vi "PieSesToAusPh.vi"(3 "error out":errorcluster, 4 "sinc":waveform(i16), 5 "Array":waveform(i16)[][](array[waveform])) -> ()   [LabVIEW 2010]
uses:
  <vilib>/Waveform/WDTOps.llb/WDT Append Waveforms DBL.vi
panel:
  out "A":i16[](array[numeric])
  out "us":sgl[](array[numeric]) format="%#.1f"
  out "size(s)":i32
  in  "index":i32
  out "Channel":string
  out "Waveform Graph":waveform(dbl)[](graph)
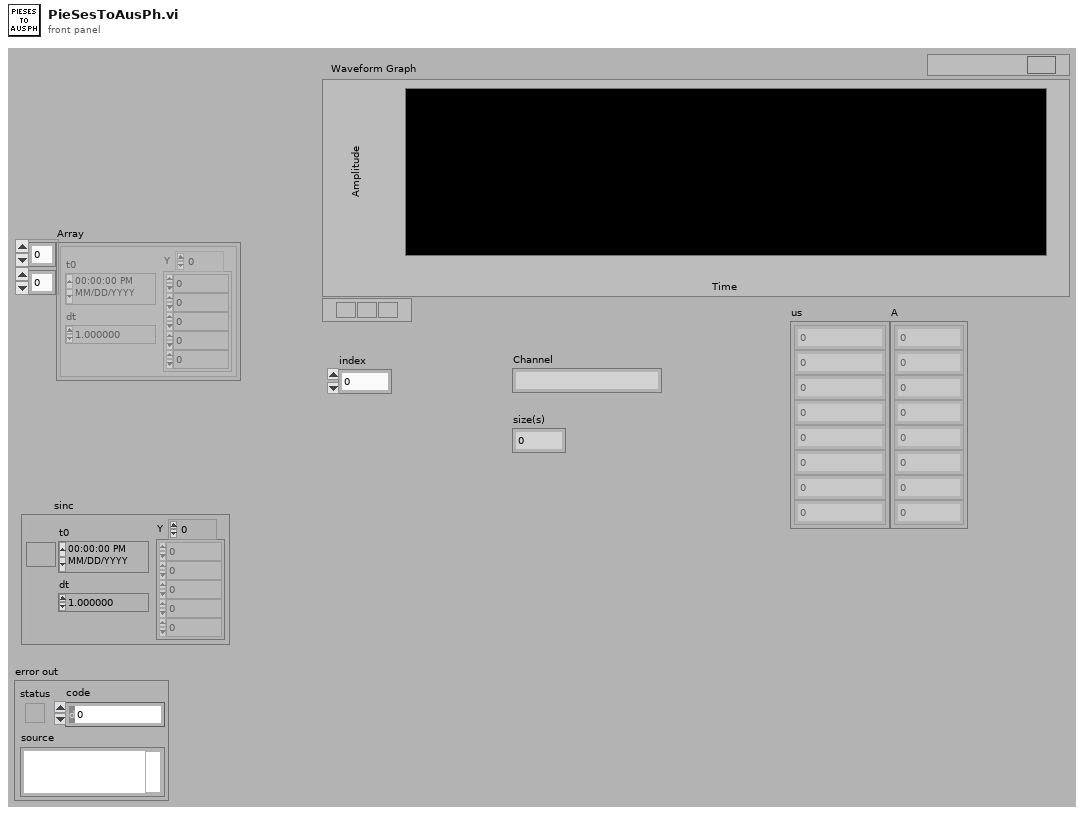
[diagram p1: front panel]
types:
  T1 = typedef "LVDateTimeRec.ctl" = cluster{"fractional second":dbl, "second":i32, "minute":i32, "hour":i32, "day of month":i32, "month":i32, "year":i32, "day of week":i32, "day of year":i32, "DST":i32}
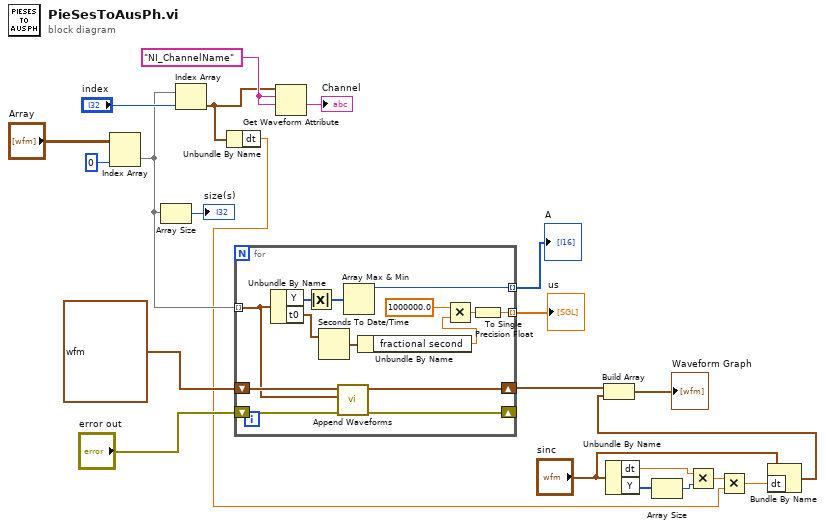
[diagram p0: block diagram]
diagram:
  w21 = "NI_ChannelName" ("name")
  n1 = Index Array(array="Array", index (col)=0 ("index (row)")) -> (element=w16:waveform(i16)[])  [unwired: 1 in]
  n2 = Array Size(array=w16) -> (size(s)=→"size(s)":i32)
  n3 = Index Array(array=w16, index="index") -> (element=w9:waveform(i16))
  n4 = Unbundle By Name(w9) -> ("dt"=w4:dbl)
  n5 = for {
    tunnel: w16 -> [w32] mode=indexing
    shift-right: [w36] -> _
    shift-left: "error out" -> [w35]
    shift-right: [w34] -> w11
    shift-left: waveform(dbl) {"t0"=timestamp(0 s since 1904-01-01), "dt"=1.0, "Y"=[]} ("waveform out") -> [w33]
    tunnel: [w29] -> w12 mode=indexing
    tunnel: [w26] -> w13 mode=indexing
    n6 = Unbundle By Name(w32) -> ("Y"=w31:i16[], "t0"=w28:timestamp)
    n7 = Absolute Value(x=w31) -> (abs(x)=w30:i16[])
    n8 = Seconds To Date/Time(time stamp (now)=w28) -> (date time rec=w27:T1)  [unwired: 1 in]
    n9 = call-poly <vilib>:"Append Waveforms.vi"("error in (no error)"=w35, "waveform B"=w32, "waveform A"=w33) -> ("error out"=w36:errorcluster, "waveform out"=w34:waveform(dbl))  [unwired: 7 in]
    n10 = Array Max & Min(array=w30) -> (max value=w29:i16)  [unwired: 3 out]
    n11 = Unbundle By Name(w27) -> ("fractional second"=w24:dbl)
    n12 = Multiply(x=1000000.0, y=w24) -> (x*y=w25:dbl)
    n13 = To Single Precision Float(number=w25) -> (single precision float=w26:sgl)
  }
  "us" <- w13
  "A" <- w12
  n14 = Get Waveform Attribute(5:w21, 6:w21, 7:w9) -> (1:→"Channel":string)  [unwired: 1 in, 3 out]
  n15 = Unbundle By Name("sinc") -> ("dt"=w6:dbl, "Y"=w8:i16[])
  n16 = Array Size(array=w8) -> (size(s)=w7:i32)
  n17 = Multiply(x=w6, y=w7) -> (x*y=w5:dbl)
  n18 = Multiply(x=w5, y=w4) -> (x*y=w2:dbl)
  n19 = Bundle By Name(cluster="sinc", "dt"=w2) -> (w1:waveform(i16))
  n20 = Build Array(w11, w1) -> (→"Waveform Graph":waveform(dbl)[])
